vi "Autonomous Independent.vi"   [LabVIEW 2015]
doc: "This VI is called when autonomous begins, and will automatically be terminated when autonomous ends. You can carry out timed or sensor driven robot movement independently without needing to return to the caller."
uses:
  BasicAuto.ctl
  AutoPortcullis.ctl
  <vilib>/Rock Robotics/WPI/Utilities/WPI_GetSetVariantRefNum.vi
  <vilib>/Rock Robotics/Network Tables/NT Read String.vi
  <vilib>/Rock Robotics/Network Tables/NT Write Numeric Array.vi
  <vilib>/Rock Robotics/Network Tables/NT Read Numeric Array.vi
  <vilib>/Rock Robotics/Network Tables/NT Read Boolean.vi
  Robot Global Data.vi
  <vilib>/Rock Robotics/WPI/RobotDrive/WPI_RobotDriveArcadeDrive_Standard(NoSaturation).vi
types:
  T1 = typedef "WPI_JoystickDevRef.ctl" = cluster{"Device":T2}
  T2 = typedef "WPI_JoystickDeviceEnum.ctl" = enum16{"USB 0", "USB 1", "USB 2", "USB 3", "USB 4", "USB 5"}
  T3 = typedef "WPI_RobotDriveDevRef.ctl" = cluster{"DevStatus":errorcluster, "Motors[]":T4[], "Square Inputs":bool, "Max Output":dbl}
  T4 = typedef "WPI_MotorControlDeviceRef.ctl" = cluster{"DeviceStatus":errorcluster, "Type":T5, "PWM":cluster{"PWM Channel":T6, "DeadBand":T7}, "CAN":cluster{"Device Number":u8, "Control Mode":T8, "Semaphore":T9, "Max Vout":dbl, "TalonSRX Control Mode":T10}, "Invert":bool}
  T5 = typedef "WPI_MotorControlType.ctl" = enum16{"PWM", "CAN", "CANTalonSRX"}
  T6 = typedef "FPGA_DIOPWMChannel.ctl" = enum8{"PWM 0", "PWM 1", "PWM 2", "PWM 3", "PWM 4", "PWM 5", "PWM 6", "PWM 7", "PWM 8", "PWM 9", "PWM MXP 0", "PWM MXP 1", "PWM MXP 2", "PWM MXP 3", "PWM MXP 4", "PWM MXP 5", "PWM MXP 6", "PWM MXP 7", "PWM MXP 8", "PWM MXP 9", "Invalid"}
  T7 = typedef "WPI_PWMDeadband.ctl" = cluster{"Name":string, "maxPositivePwm":i32, "minPositivePwm":i32, "centerPwm":i32, "maxNegativePwm":i32, "minNegativePwm":i32, "angularRange":u16}
  T8 = typedef "WPI_CANJaguar_ControlMode.ctl" = enum8{"Percent VBus", "Current", "Speed", "Position", "Voltage"}
  T9 = typedef "Semaphore RefNum" = refnum<k1>
  T10 = typedef "WPI_CANTalonSRX_APIControlMode.ctl" = enum8{"Percent VBus", "Speed", "Position", "Slave", "Unchanged / Invalid", "Voltage Compensation", "Current", "Motion Profile"}
  T11 = typedef "WPI_DigitalInputDevRef.ctl" = cluster{"DevStatus":errorcluster, "DIO Channel":T12}
  T12 = typedef "FPGA_DIOChannel.ctl" = enum8{"DIO 0", "DIO 1", "DIO 2", "DIO 3", "DIO 4", "DIO 5", "DIO 6", "DIO 7", "DIO 8", "DIO 9", "DIO MXP 0", "DIO MXP 1", "DIO MXP 2", "DIO MXP 3", "DIO MXP 4", "DIO MXP 5", "DIO MXP 6", "DIO MXP 7", "DIO MXP 8", "DIO MXP 9", "DIO MXP 10", "DIO MXP 11", "DIO MXP 12", "DIO MXP 13", "DIO MXP 14", "DIO MXP 15", "Invalid"}
  T13 = cluster{dbl, "RobotDriveDevRef":T3, "Numeric Array":dbl[], "Boolean":bool}
  T14 = cluster{"DigitalInputDevRef":T11, "DigitalInputDevRef":T11, "MotorControlDevRef":T4}
  T15 = typedef "BasicAuto.ctl" = enum16{"Idle", "Approach", "Breach", "Travel", "Turn", "AutoTarget", "Stop"}
  T16 = typedef "AutoPortcullis.ctl" = enum16{"Idle", "Approach", "Rest", "ArmDown", "ReverseBall", "Breach", "Travel", "Stop"}
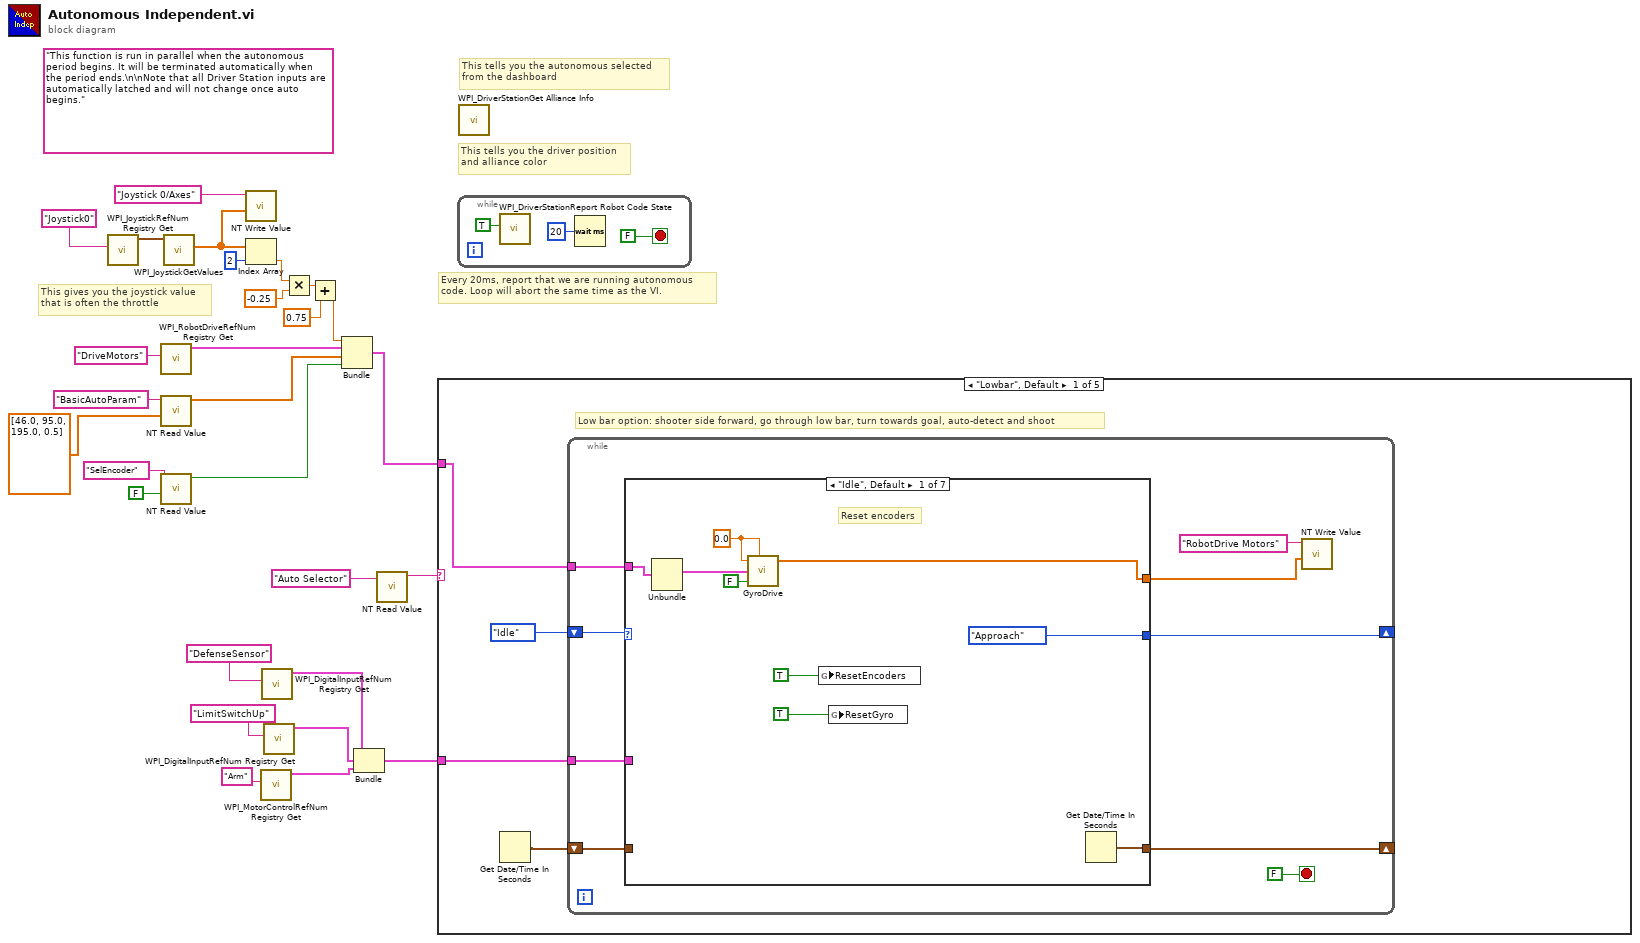
[diagram p0: block diagram]
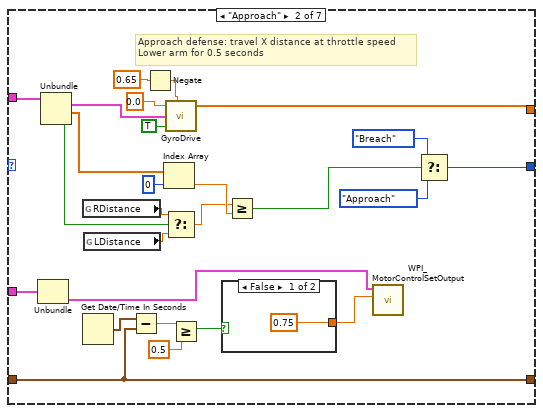
[diagram p2: hidden frame]
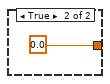
[diagram p3: hidden frame]
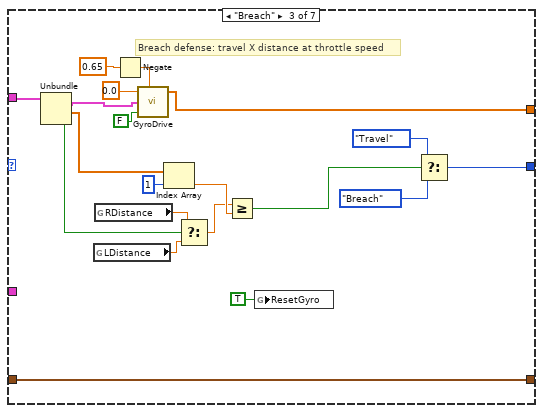
[diagram p4: hidden frame]
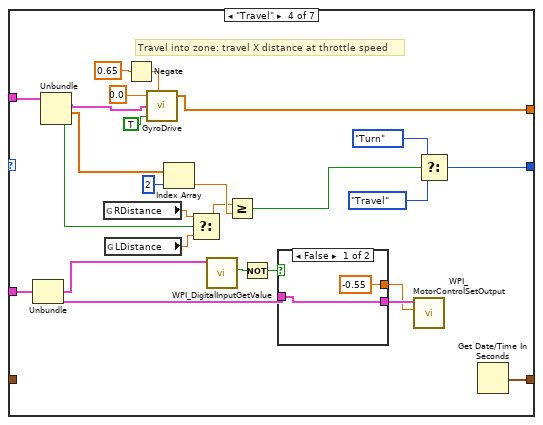
[diagram p5: hidden frame]
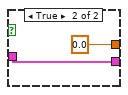
[diagram p6: hidden frame]
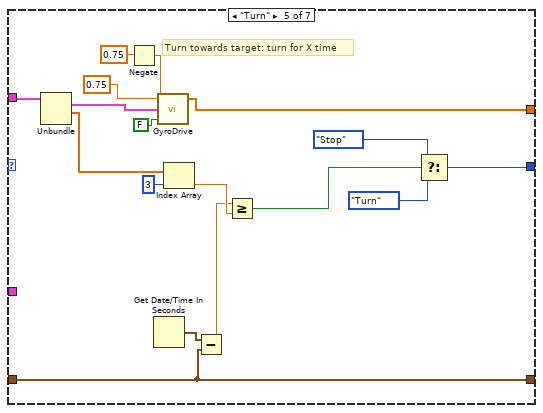
[diagram p7: hidden frame]
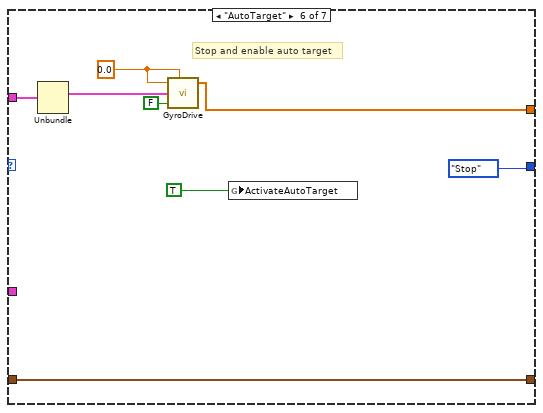
[diagram p8: hidden frame]
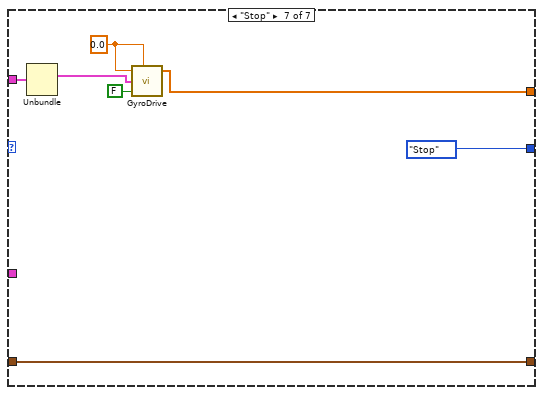
[diagram p9: hidden frame]
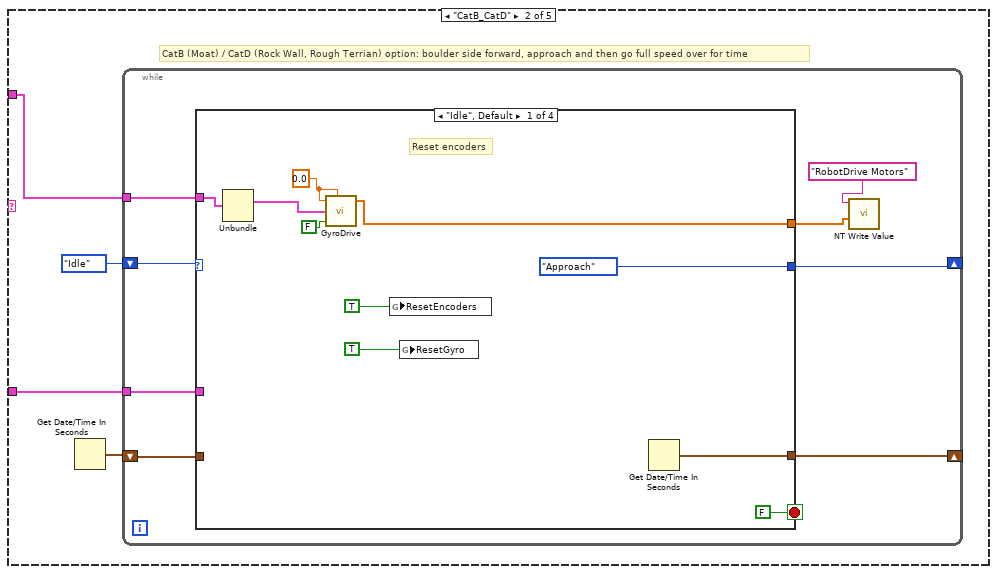
[diagram p10: hidden frame]
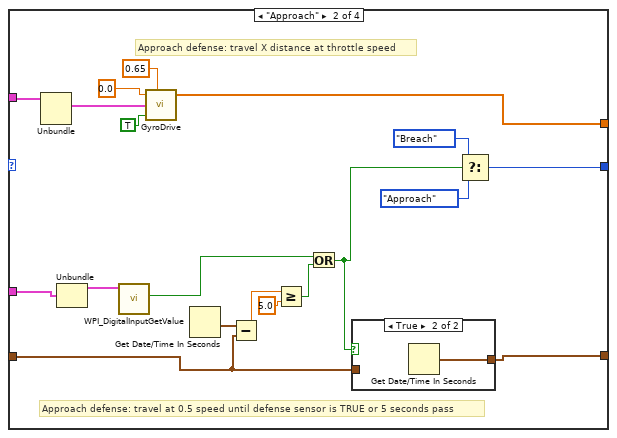
[diagram p11: hidden frame]
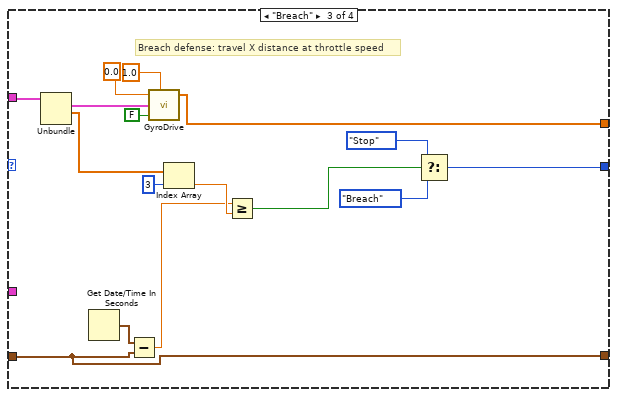
[diagram p13: hidden frame]
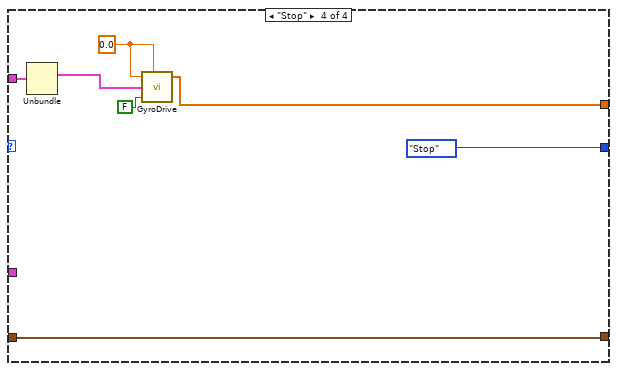
[diagram p14: hidden frame]
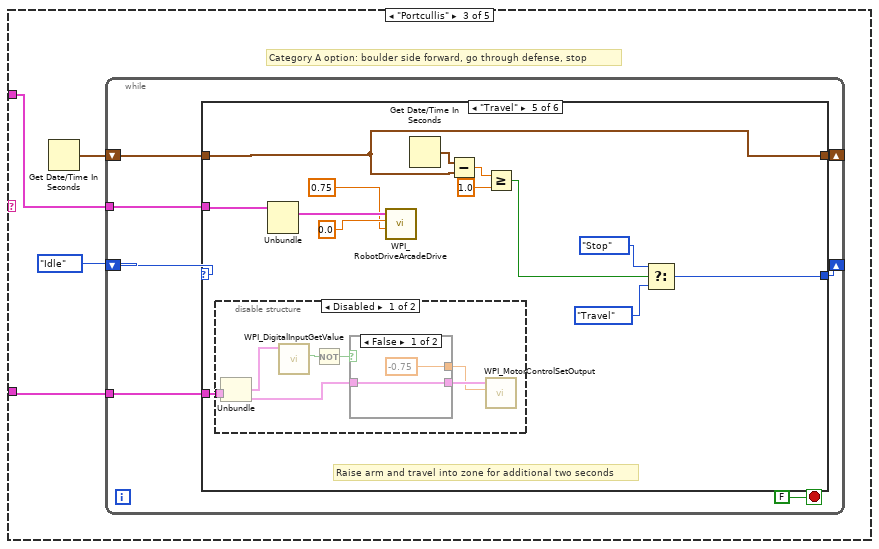
[diagram p15: hidden frame]
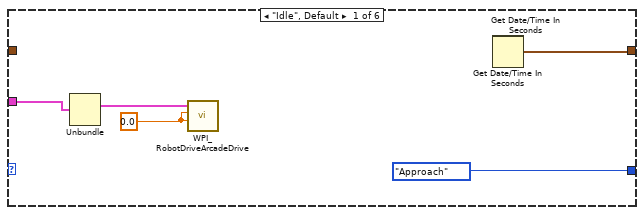
[diagram p16: hidden frame]
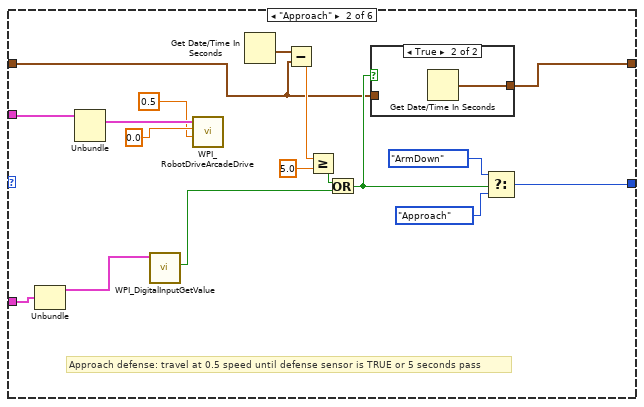
[diagram p17: hidden frame]
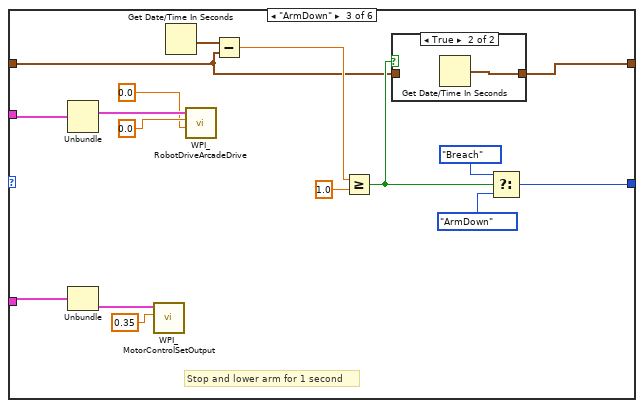
[diagram p19: hidden frame]
diagram:
  (unwired) "This function is run in parallel when the autonomous period begins. It will be terminated automatically when the period ends.\n\nNote that all Driver Station inputs are automatically latched and will not change once auto begins."
  # "This tells you the autonomous selected\nfrom the dashboard"
  # "Every 20ms, report that we are running autonomous\ncode. Loop will abort the same time as the VI."
  # "This gives you the joystick value\nthat is often the throttle"
  # "This tells you the driver position\nand alliance color"
  n1 = call <vilib>:"WPI_JoystickRefNum Registry Get.vi"("refnum name"="Joystick0") -> ("JoystickDevRef"=w27:T1)  [unwired: 1 in, 9 out]
  n2 = call <vilib>:"WPI_RobotDriveRefNum Registry Get.vi"("refnum name"="DriveMotors") -> ("RobotDriveDevRef"=w20:T3)  [unwired: 9 in, 1 out]
  n3 = call-poly <vilib>:"NT Read Value.vi"("Default Value"=dbl[] [46.0, 95.0, 195.0, 0.5], "Name"="BasicAutoParam") -> ("Numeric Array"=w17:dbl[])  [unwired: 8 in, 1 out]
  n4 = call-poly <vilib>:"NT Read Value.vi"("Default Value"=FALSE, "Name"="SelEncoder") -> ("Boolean"=w13:bool)  [unwired: 8 in, 1 out]
  n5 = call <vilib>:"WPI_JoystickGetValues.vi"("JoystickDevRef"=w27) -> ("Axes"=w23:dbl[])  [unwired: 6 in, 4 out]
  n6 = call-poly <vilib>:"NT Write Value.vi"("Numeric Array"=w23, "Name"="Joystick 0/Axes") -> ()  [unwired: 9 in, 1 out]
  n7 = Index Array(array=w23, index=2) -> (element=w9:dbl)
  n8 = call <vilib>:"WPI_MotorControlRefNum Registry Get.vi"("refnum name"="Arm") -> ("MotorControlDevRef"=w2:T4)  [unwired: 9 in, 1 out]
  n9 = call <vilib>:"WPI_DigitalInputRefNum Registry Get.vi"("refnum name"="DefenseSensor") -> ("DigitalInputDevRef"=w4:T11)  [unwired: 9 in, 1 out]
  n10 = call <vilib>:"WPI_DigitalInputRefNum Registry Get.vi"("refnum name"="LimitSwitchUp") -> ("DigitalInputDevRef"=w3:T11)  [unwired: 9 in, 1 out]
  n11 = Multiply(x=w9, y=-0.25) -> (x*y=w11:dbl)
  n12 = Add(x=w11, y=0.75) -> (x+y=w8:dbl)
  n13 = Bundle(w8, "RobotDriveDevRef"=w20, "Numeric Array"=w17, "Boolean"=w13) -> (w19:T13)  [unwired: 1 in]
  n14 = Bundle("DigitalInputDevRef"=w4, "DigitalInputDevRef"=w3, "MotorControlDevRef"=w2) -> (w1:T14)  [unwired: 1 in]
  n15 = call-poly <vilib>:"NT Read Value.vi"("Name"="Auto Selector") -> ("String"=w24:string)  [unwired: 9 in, 1 out]
  n16 = case shown="\"Lowbar\", Default" w24 {
    tunnel: w19 -> [w31 w163 w230 w327 w452]
    tunnel: w1 -> [w30 w162 w227 w324 w451]
    frame "Lowbar", Default {
      # "Low bar option: shooter side forward, go through low bar, turn towards goal, auto-detect and shoot"
      n17 = Get Date/Time In Seconds() -> (seconds since 1Jan1904=w29:timestamp)
      n18 = while {
        shift-right: [w39] -> _
        shift-left: BasicAuto."Idle" ("BasicAuto") -> [w41]
        tunnel: w31 -> [w38]
        shift-right: [w36] -> _
        shift-left: w29 -> [w37]
        tunnel: w30 -> [w35]
        stop <- FALSE stop-if-true
        n19 = case shown="\"Idle\", Default" w41 {
          tunnel: [BasicAuto."Approach" ("BasicAuto") w70 w92 w118 w139 BasicAuto."Stop" ("BasicAuto") BasicAuto."Stop" ("BasicAuto")] -> w39
          tunnel: w38 -> [w48 w76 w98 w124 w145 w152 w158]
          tunnel: [w47 w63 w86 w107 w136 w150 w159] -> w36
          tunnel: w37 -> [_ w63 w86 _ w136 w150 w159]
          tunnel: w35 -> [_ w59 _ w112 _ _ _]
          tunnel: [w44 w52 w80 w99 w129 w146 w155] -> w33
          frame "Idle", Default {
            w46 = 0.0 ("X axis value")
            # "Reset encoders"
            n20 = Unbundle(w48) -> ("RobotDriveDevRef"=w45:T3)  [unwired: 3 out]
            n21 = call "GyroDrive.vi"("X axis value"=w46, "Y axis value"=w46, "RobotDriveDevRef_In"=w45, "Use gyro"=FALSE) -> ("Motor Values"=w44:dbl[])  [unwired: 1 in, 2 out]
            n22 = global write "Robot Global Data.vi" "ResetEncoders"(TRUE) -> ()
            n23 = global write "Robot Global Data.vi" "ResetGyro"(TRUE) -> ()
            n24 = Get Date/Time In Seconds() -> (seconds since 1Jan1904=w47:timestamp)
          }
          frame "Approach" {
            # "Approach defense: travel X distance at throttle speed\nLower arm for 0.5 seconds"
            n25 = Unbundle(w59) -> ("MotorControlDevRef"=w57:T4)  [unwired: 2 out]
            n26 = Unbundle(w76) -> ("RobotDriveDevRef"=w53:T3, "Numeric Array"=w75:dbl[], "Boolean"=w68:bool)  [unwired: 1 out]
            n27 = global read "Robot Global Data.vi" "RDistance"() -> (w66:dbl)
            n28 = Get Date/Time In Seconds() -> (seconds since 1Jan1904=w64:timestamp)
            n29 = global read "Robot Global Data.vi" "LDistance"() -> (w67:dbl)
            n30 = Subtract(x=w64, y=w63) -> (x-y=w62:dbl)
            n31 = Negate(x=0.65 ("X axis value")) -> (-x=w55:dbl)
            n32 = Index Array(array=w75, index=0) -> (element=w74:dbl)
            n33 = call "GyroDrive.vi"("X axis value"=0.0, "Y axis value"=w55, "RobotDriveDevRef_In"=w53, "Use gyro"=TRUE) -> ("Motor Values"=w52:dbl[])  [unwired: 1 in, 2 out]
            n34 = Select(t=w66, s=w68, f=w67) -> (s? t:f=w65:dbl)
            n35 = Greater Or Equal?(x=w62, y=0.5) -> (x >= y?=w60:bool)
            n36 = case shown="False" w60 {
              tunnel: [0.75 0.0 ("Output")] -> w56
              frame False {
              }
              frame True {
              }
            }
            n37 = Greater Or Equal?(x=w65, y=w74) -> (x >= y?=w73:bool)
            n38 = call <vilib>:"WPI_MotorControlSetOutput.vi"("Output"=w56, "MotorControlDevRef"=w57) -> ()  [unwired: 7 in, 3 out]
            n39 = Select(t=BasicAuto."Breach" ("BasicAuto"), s=w73, f=BasicAuto."Approach" ("BasicAuto")) -> (s? t:f=w70:T15)
          }
          frame "Breach" {
            # "Breach defense: travel X distance at throttle speed"
            n40 = Unbundle(w98) -> ("RobotDriveDevRef"=w82:T3, "Numeric Array"=w97:dbl[], "Boolean"=w89:bool)  [unwired: 1 out]
            n41 = global read "Robot Global Data.vi" "LDistance"() -> (w88:dbl)
            n42 = global read "Robot Global Data.vi" "RDistance"() -> (w90:dbl)
            n43 = Negate(x=0.65 ("X axis value")) -> (-x=w84:dbl)
            n44 = call "GyroDrive.vi"("X axis value"=0.0, "Y axis value"=w84, "RobotDriveDevRef_In"=w82, "Use gyro"=FALSE) -> ("Motor Values"=w80:dbl[])  [unwired: 1 in, 2 out]
            n45 = Index Array(array=w97, index=1) -> (element=w96:dbl)
            n46 = Select(t=w90, s=w89, f=w88) -> (s? t:f=w87:dbl)
            n47 = Greater Or Equal?(x=w87, y=w96) -> (x >= y?=w95:bool)
            n48 = global write "Robot Global Data.vi" "ResetGyro"(TRUE ("ResetGyro")) -> ()
            n49 = Select(t=BasicAuto."Travel" ("BasicAuto"), s=w95, f=BasicAuto."Breach" ("BasicAuto")) -> (s? t:f=w92:T15)
          }
          frame "Travel" {
            # "Travel into zone: travel X distance at throttle speed"
            n50 = Unbundle(w112) -> ("DigitalInputDevRef"=w109:T11, "MotorControlDevRef"=w105:T4)  [unwired: 1 out]
            n51 = Unbundle(w124) -> ("RobotDriveDevRef"=w101:T3, "Numeric Array"=w123:dbl[], "Boolean"=w114:bool)  [unwired: 1 out]
            n52 = global read "Robot Global Data.vi" "RDistance"() -> (w116:dbl)
            n53 = global read "Robot Global Data.vi" "LDistance"() -> (w115:dbl)
            n54 = Negate(x=0.65 ("X axis value")) -> (-x=w103:dbl)
            n55 = call "GyroDrive.vi"("X axis value"=0.0, "Y axis value"=w103, "RobotDriveDevRef_In"=w101, "Use gyro"=TRUE) -> ("Motor Values"=w99:dbl[])  [unwired: 1 in, 2 out]
            n56 = Index Array(array=w123, index=2) -> (element=w122:dbl)
            n57 = Select(t=w116, s=w114, f=w115) -> (s? t:f=w113:dbl)
            n58 = call <vilib>:"WPI_DigitalInputGetValue.vi"("DigitalInputDevRef"=w109) -> ("Value"=w110:bool)  [unwired: 8 in, 2 out]
            n59 = Greater Or Equal?(x=w113, y=w122) -> (x >= y?=w121:bool)
            n60 = Not(x=w110) -> (.not. x?=w111:bool)
            n61 = case shown="False" w111 {
              tunnel: [w126 w128] -> w106
              tunnel: w105 -> [w126 w128]
              tunnel: [-0.55 ("Output") 0.0 ("Output")] -> w104
              frame False {
              }
              frame True {
              }
            }
            n62 = call <vilib>:"WPI_MotorControlSetOutput.vi"("Output"=w104, "MotorControlDevRef"=w106) -> ()  [unwired: 7 in, 3 out]
            n63 = Select(t=BasicAuto."Turn" ("BasicAuto"), s=w121, f=BasicAuto."Travel" ("BasicAuto")) -> (s? t:f=w118:T15)
            n64 = Get Date/Time In Seconds() -> (seconds since 1Jan1904=w107:timestamp)
          }
          frame "Turn" {
            # "Turn towards target: turn for X time"
            n65 = Unbundle(w145) -> ("RobotDriveDevRef"=w133:T3, "Numeric Array"=w144:dbl[])  [unwired: 2 out]
            n66 = Negate(x=0.75 ("y")) -> (-x=w132:dbl)
            n67 = Get Date/Time In Seconds() -> (seconds since 1Jan1904=w137:timestamp)
            n68 = call "GyroDrive.vi"("X axis value"=0.75, "Y axis value"=w132, "RobotDriveDevRef_In"=w133, "Use gyro"=FALSE) -> ("Motor Values"=w129:dbl[])  [unwired: 1 in, 2 out]
            n69 = Index Array(array=w144, index=3) -> (element=w143:dbl)
            n70 = Subtract(x=w137, y=w136) -> (x-y=w135:dbl)
            n71 = Greater Or Equal?(x=w135, y=w143) -> (x >= y?=w142:bool)
            n72 = Select(t=BasicAuto."Stop" ("BasicAuto"), s=w142, f=BasicAuto."Turn" ("BasicAuto")) -> (s? t:f=w139:T15)
          }
          frame "AutoTarget" {
            w148 = 0.0 ("X axis value")
            # "Stop and enable auto target"
            n73 = Unbundle(w152) -> ("RobotDriveDevRef"=w149:T3)  [unwired: 3 out]
            n74 = call "GyroDrive.vi"("X axis value"=w148, "Y axis value"=w148, "RobotDriveDevRef_In"=w149, "Use gyro"=FALSE) -> ("Motor Values"=w146:dbl[])  [unwired: 1 in, 2 out]
            n75 = global write "Robot Global Data.vi" "ActivateAutoTarget"(TRUE ("ActivateAutoTarget")) -> ()
          }
          frame "Stop" {
            w157 = 0.0 ("X axis value")
            n76 = Unbundle(w158) -> ("RobotDriveDevRef"=w156:T3)  [unwired: 3 out]
            n77 = call "GyroDrive.vi"("X axis value"=w157, "Y axis value"=w157, "RobotDriveDevRef_In"=w156, "Use gyro"=FALSE) -> ("Motor Values"=w155:dbl[])  [unwired: 1 in, 2 out]
          }
        }
        n78 = call-poly <vilib>:"NT Write Value.vi"("Numeric Array"=w33, "Name"="RobotDrive Motors") -> ()  [unwired: 9 in, 1 out]
      }
    }
    frame "CatB_CatD" {
      # "CatB (Moat) / CatD (Rock Wall, Rough Terrian) option: boulder side forward, approach and then go full speed over for time"
      n79 = Get Date/Time In Seconds() -> (seconds since 1Jan1904=w161:timestamp)
      n80 = while {
        shift-right: [w171] -> _
        shift-left: BasicAuto."Idle" ("BasicAuto") -> [w173]
        tunnel: w163 -> [w170]
        tunnel: w162 -> [w169]
        shift-right: [w168] -> _
        shift-left: w161 -> [w167]
        stop <- FALSE stop-if-true
        n81 = case shown="\"Idle\", Default" w173 {
          tunnel: [BasicAuto."Approach" ("BasicAuto") w198 w213 BasicAuto."Stop" ("BasicAuto")] -> w171
          tunnel: w170 -> [w180 w201 w219 w225]
          tunnel: w169 -> [_ w192 _ _]
          tunnel: [w179 w190 w210 w224] -> w168
          tunnel: w167 -> [_ w189 w210 w224]
          tunnel: [w174 w194 w205 w221] -> w165
          frame "Idle", Default {
            w176 = 0.0 ("X axis value")
            # "Reset encoders"
            n82 = Unbundle(w180) -> ("RobotDriveDevRef"=w177:T3)  [unwired: 3 out]
            n83 = call "GyroDrive.vi"("X axis value"=w176, "Y axis value"=w176, "RobotDriveDevRef_In"=w177, "Use gyro"=FALSE) -> ("Motor Values"=w174:dbl[])  [unwired: 1 in, 2 out]
            n84 = global write "Robot Global Data.vi" "ResetEncoders"(TRUE) -> ()
            n85 = global write "Robot Global Data.vi" "ResetGyro"(TRUE ("ResetGyro")) -> ()
            n86 = Get Date/Time In Seconds() -> (seconds since 1Jan1904=w179:timestamp)
          }
          frame "Approach" {
            # "Approach defense: travel at 0.5 speed until defense sensor is TRUE or 5 seconds pass"
            # "Approach defense: travel X distance at throttle speed"
            n87 = Unbundle(w201) -> ("RobotDriveDevRef"=w197:T3)  [unwired: 3 out]
            n88 = Unbundle(w192) -> ("DigitalInputDevRef"=w193:T11)  [unwired: 2 out]
            n89 = call <vilib>:"WPI_DigitalInputGetValue.vi"("DigitalInputDevRef"=w193) -> ("Value"=w186:bool)  [unwired: 8 in, 2 out]
            n90 = call "GyroDrive.vi"("X axis value"=0.0, "Y axis value"=0.65 ("X axis value"), "RobotDriveDevRef_In"=w197, "Use gyro"=TRUE) -> ("Motor Values"=w194:dbl[])  [unwired: 1 in, 2 out]
            n91 = Get Date/Time In Seconds() -> (seconds since 1Jan1904=w191:timestamp)
            n92 = Subtract(x=w191, y=w189) -> (x-y=w187:dbl)
            n93 = Greater Or Equal?(x=w187, y=5.0) -> (x >= y?=w185:bool)
            n94 = Or(x=w186, y=w185) -> (x .or. y?=w184:bool)
            n95 = case shown="True" w184 {
              tunnel: [w202 w203] -> w190
              tunnel: w189 -> [w202 _]
              frame False {
              }
              frame True {
                n96 = Get Date/Time In Seconds() -> (seconds since 1Jan1904=w203:timestamp)
              }
            }
            n97 = Select(t=BasicAuto."Breach" ("BasicAuto"), s=w184, f=BasicAuto."Approach" ("BasicAuto")) -> (s? t:f=w198:T15)
          }
          frame "Breach" {
            # "Breach defense: travel X distance at throttle speed"
            n98 = Unbundle(w219) -> ("RobotDriveDevRef"=w206:T3, "Numeric Array"=w218:dbl[])  [unwired: 2 out]
            n99 = Get Date/Time In Seconds() -> (seconds since 1Jan1904=w211:timestamp)
            n100 = Subtract(x=w211, y=w210) -> (x-y=w209:dbl)
            n101 = call "GyroDrive.vi"("X axis value"=0.0, "Y axis value"=1.0 ("X axis value"), "RobotDriveDevRef_In"=w206, "Use gyro"=FALSE) -> ("Motor Values"=w205:dbl[])  [unwired: 1 in, 2 out]
            n102 = Index Array(array=w218, index=3) -> (element=w217:dbl)
            n103 = Greater Or Equal?(x=w209, y=w217) -> (x >= y?=w216:bool)
            n104 = Select(t=BasicAuto."Stop" ("BasicAuto"), s=w216, f=BasicAuto."Breach" ("BasicAuto")) -> (s? t:f=w213:T15)
          }
          frame "Stop" {
            w223 = 0.0 ("X axis value")
            n105 = Unbundle(w225) -> ("RobotDriveDevRef"=w222:T3)  [unwired: 3 out]
            n106 = call "GyroDrive.vi"("X axis value"=w223, "Y axis value"=w223, "RobotDriveDevRef_In"=w222, "Use gyro"=FALSE) -> ("Motor Values"=w221:dbl[])  [unwired: 1 in, 2 out]
          }
        }
        n107 = call-poly <vilib>:"NT Write Value.vi"("Numeric Array"=w165, "Name"="RobotDrive Motors") -> ()  [unwired: 9 in, 1 out]
      }
    }
    frame "Portcullis" {
      # "Category A option: boulder side forward, go through defense, stop"
      n108 = Get Date/Time In Seconds() -> (seconds since 1Jan1904=w228:timestamp)
      n109 = while {
        shift-right: [w235] -> _
        shift-left: AutoPortcullis."Idle" ("AutoPortcullis") -> [w237]
        tunnel: w230 -> [w234]
        shift-right: [w232] -> _
        shift-left: w228 -> [w233]
        tunnel: w227 -> [w231]
        stop <- FALSE stop-if-true
        n110 = case shown="\"Travel\"" w237 {
          tunnel: [AutoPortcullis."Approach" ("AutoPortcullis") w257 w276 w290 w305 AutoPortcullis."Stop" ("AutoPortcullis")] -> w235
          tunnel: w234 -> [w242 w259 w268 w292 w307 w323]
          tunnel: w233 -> [_ w245 w265 w280 w299 w320]
          tunnel: [w238 w246 w267 w281 w299 w320] -> w232
          tunnel: w231 -> [_ w244 w264 _ w295 _]
          frame "Idle", Default {
            w240 = 0.0 ("X axis value")
            n111 = Unbundle(w242) -> ("RobotDriveDevRef"=w241:T3)  [unwired: 3 out]
            n112 = call-poly <vilib>:"WPI_RobotDriveArcadeDrive.vi"("Y axis value"=w240, "X axis value"=w240, "RobotDriveDevRef"=w241) -> ()  [unwired: 6 in, 3 out]
            n113 = Get Date/Time In Seconds() -> (seconds since 1Jan1904=w238:timestamp)
            n114 = Get Date/Time In Seconds() -> ()  [unwired: 1 out]
          }
          frame "Approach" {
            # "Approach defense: travel at 0.5 speed until defense sensor is TRUE or 5 seconds pass"
            n115 = Unbundle(w244) -> ("DigitalInputDevRef"=w243:T11)  [unwired: 2 out]
            n116 = Unbundle(w259) -> ("RobotDriveDevRef"=w258:T3)  [unwired: 3 out]
            n117 = call <vilib>:"WPI_DigitalInputGetValue.vi"("DigitalInputDevRef"=w243) -> ("Value"=w248:bool)  [unwired: 8 in, 2 out]
            n118 = call-poly <vilib>:"WPI_RobotDriveArcadeDrive.vi"("Y axis value"=0.5 ("X axis value"), "X axis value"=0.0, "RobotDriveDevRef"=w258) -> ()  [unwired: 6 in, 3 out]
            n119 = Get Date/Time In Seconds() -> (seconds since 1Jan1904=w252:timestamp)
            n120 = Subtract(x=w252, y=w245) -> (x-y=w251:dbl)
            n121 = Greater Or Equal?(x=w251, y=5.0) -> (x >= y?=w249:bool)
            n122 = Or(x=w249, y=w248) -> (x .or. y?=w247:bool)
            n123 = case shown="True" w247 {
              tunnel: [w260 w261] -> w246
              tunnel: w245 -> [w260 _]
              frame False {
              }
              frame True {
                n124 = Get Date/Time In Seconds() -> (seconds since 1Jan1904=w261:timestamp)
              }
            }
            n125 = Select(t=AutoPortcullis."ArmDown" ("AutoPortcullis"), s=w247, f=AutoPortcullis."Approach" ("AutoPortcullis")) -> (s? t:f=w257:T16)
          }
          frame "ArmDown" {
            # "Stop and lower arm for 1 second"
            n126 = Unbundle(w268) -> ("RobotDriveDevRef"=w271:T3)  [unwired: 3 out]
            n127 = Unbundle(w264) -> ("MotorControlDevRef"=w263:T4)  [unwired: 2 out]
            n128 = call <vilib>:"WPI_MotorControlSetOutput.vi"("Output"=0.35, "MotorControlDevRef"=w263) -> ()  [unwired: 7 in, 3 out]
            n129 = Get Date/Time In Seconds() -> (seconds since 1Jan1904=w277:timestamp)
            n130 = call-poly <vilib>:"WPI_RobotDriveArcadeDrive.vi"("Y axis value"=0.0 ("X axis value"), "X axis value"=0.0, "RobotDriveDevRef"=w271) -> ()  [unwired: 6 in, 3 out]
            n131 = Subtract(x=w277, y=w265) -> (x-y=w275:dbl)
            n132 = Greater Or Equal?(x=w275, y=1.0) -> (x >= y?=w266:bool)
            n133 = case shown="True" w266 {
              tunnel: [w278 w279] -> w267
              tunnel: w265 -> [w278 _]
              frame False {
              }
              frame True {
                n134 = Get Date/Time In Seconds() -> (seconds since 1Jan1904=w279:timestamp)
              }
            }
            n135 = Select(t=AutoPortcullis."Breach" ("AutoPortcullis"), s=w266, f=AutoPortcullis."ArmDown" ("AutoPortcullis")) -> (s? t:f=w276:T16)
          }
          frame "Breach" {
            # "Breach defense: start moving forward at higher speed"
            n136 = Unbundle(w292) -> ("RobotDriveDevRef"=w291:T3)  [unwired: 3 out]
            n137 = call-poly <vilib>:"WPI_RobotDriveArcadeDrive.vi"("Y axis value"=0.75 ("X axis value"), "X axis value"=0.0, "RobotDriveDevRef"=w291) -> ()  [unwired: 6 in, 3 out]
            n138 = Get Date/Time In Seconds() -> (seconds since 1Jan1904=w288:timestamp)
            n139 = Subtract(x=w288, y=w280) -> (x-y=w287:dbl)
            n140 = Greater Or Equal?(x=w287, y=2.0) -> (x >= y?=w282:bool)
            n141 = case shown="True" w282 {
              tunnel: [w293 w294] -> w281
              tunnel: w280 -> [w293 _]
              frame False {
              }
              frame True {
                n142 = Get Date/Time In Seconds() -> (seconds since 1Jan1904=w294:timestamp)
              }
            }
            n143 = Select(t=AutoPortcullis."Travel" ("AutoPortcullis"), s=w282, f=AutoPortcullis."Breach" ("AutoPortcullis")) -> (s? t:f=w290:T16)
          }
          frame "Travel" {
            # "Raise arm and travel into zone for additional two seconds"
            n144 = disable-structure shown="Disabled" {
              disable-tunnel: w295 -> [w312 _]
              frame Disabled {
                n145 = Unbundle(w312) -> ("DigitalInputDevRef"=w311:T11, "MotorControlDevRef"=w310:T4)  [unwired: 1 out]
                n146 = call <vilib>:"WPI_DigitalInputGetValue.vi"("DigitalInputDevRef"=w311) -> ("Value"=w313:bool)  [unwired: 8 in, 2 out]
                n147 = Not(x=w313) -> (.not. x?=w314:bool)
                n148 = case shown="False" w314 {
                  tunnel: w310 -> [w316 w318]
                  tunnel: [w316 w318] -> w309
                  tunnel: [-0.75 ("Output") 0.0 ("Output")] -> w308
                  frame False {
                  }
                  frame True {
                  }
                }
                n149 = call <vilib>:"WPI_MotorControlSetOutput.vi"("Output"=w308, "MotorControlDevRef"=w309) -> ()  [unwired: 7 in, 3 out]
              }
              frame Enabled {
              }
            }
            n150 = Unbundle(w307) -> ("RobotDriveDevRef"=w306:T3)  [unwired: 3 out]
            n151 = call-poly <vilib>:"WPI_RobotDriveArcadeDrive.vi"("Y axis value"=0.75 ("X axis value"), "X axis value"=0.0, "RobotDriveDevRef"=w306) -> ()  [unwired: 6 in, 3 out]
            n152 = Get Date/Time In Seconds() -> (seconds since 1Jan1904=w303:timestamp)
            n153 = Subtract(x=w303, y=w299) -> (x-y=w302:dbl)
            n154 = Greater Or Equal?(x=w302, y=1.0) -> (x >= y?=w300:bool)
            n155 = Select(t=AutoPortcullis."Stop" ("AutoPortcullis"), s=w300, f=AutoPortcullis."Travel" ("AutoPortcullis")) -> (s? t:f=w305:T16)
          }
          frame "Stop" {
            w321 = 0.0 ("X axis value")
            n156 = Unbundle(w323) -> ("RobotDriveDevRef"=w322:T3)  [unwired: 3 out]
            n157 = call-poly <vilib>:"WPI_RobotDriveArcadeDrive.vi"("Y axis value"=w321, "X axis value"=w321, "RobotDriveDevRef"=w322) -> ()  [unwired: 6 in, 3 out]
          }
        }
      }
    }
    frame "Cheval" {
      # "Category A option: boulder side forward, go through defense, stop"
      n158 = Get Date/Time In Seconds() -> (seconds since 1Jan1904=w325:timestamp)
      n159 = while {
        shift-right: [w334] -> _
        shift-left: AutoPortcullis."Idle" ("AutoPortcullis") -> [w336]
        tunnel: w327 -> [w333]
        shift-right: [w331] -> _
        shift-left: w325 -> [w332]
        tunnel: w324 -> [w330]
        stop <- FALSE stop-if-true
        n160 = case shown="\"Idle\", Default" w336 {
          tunnel: [AutoPortcullis."Approach" ("AutoPortcullis") w362 w378 w397 w414 w437 AutoPortcullis."Stop" ("AutoPortcullis")] -> w334
          tunnel: w333 -> [w344 w363 w379 w392 w415 w438 w449]
          tunnel: w332 -> [_ w352 w371 w389 w407 w432 w448]
          tunnel: [w342 w353 w372 w391 w408 w432 w448] -> w331
          tunnel: w330 -> [_ w351 _ w388 _ w429 _]
          tunnel: [w338 w346 w367 w383 w401 w419 w443] -> w328
          frame "Idle", Default {
            w340 = 0.0 ("X axis value")
            n161 = Unbundle(w344) -> ("RobotDriveDevRef"=w341:T3)  [unwired: 3 out]
            n162 = global write "Robot Global Data.vi" "ResetGyro"(TRUE ("ResetGyro")) -> ()
            n163 = call "GyroDrive.vi"("X axis value"=w340, "Y axis value"=w340, "RobotDriveDevRef_In"=w341, "Use gyro"=FALSE) -> ("Motor Values"=w338:dbl[])  [unwired: 1 in, 2 out]
            n164 = Get Date/Time In Seconds() -> (seconds since 1Jan1904=w342:timestamp)
            n165 = Get Date/Time In Seconds() -> ()  [unwired: 1 out]
          }
          frame "Approach" {
            # "Approach defense: travel at 0.5 speed until defense sensor is TRUE or 5 seconds pass"
            n166 = Unbundle(w351) -> ("DigitalInputDevRef"=w350:T11)  [unwired: 2 out]
            n167 = Unbundle(w363) -> ("RobotDriveDevRef"=w347:T3)  [unwired: 3 out]
            n168 = call <vilib>:"WPI_DigitalInputGetValue.vi"("DigitalInputDevRef"=w350) -> ("Value"=w355:bool)  [unwired: 8 in, 2 out]
            n169 = call "GyroDrive.vi"("X axis value"=0.0, "Y axis value"=0.55 ("X axis value"), "RobotDriveDevRef_In"=w347, "Use gyro"=TRUE) -> ("Motor Values"=w346:dbl[])  [unwired: 1 in, 2 out]
            n170 = Get Date/Time In Seconds() -> (seconds since 1Jan1904=w359:timestamp)
            n171 = Subtract(x=w359, y=w352) -> (x-y=w358:dbl)
            n172 = Greater Or Equal?(x=w358, y=5.0) -> (x >= y?=w356:bool)
            n173 = Or(x=w356, y=w355) -> (x .or. y?=w354:bool)
            n174 = case shown="True" w354 {
              tunnel: [w364 w365] -> w353
              tunnel: w352 -> [w364 _]
              frame False {
              }
              frame True {
                n175 = Get Date/Time In Seconds() -> (seconds since 1Jan1904=w365:timestamp)
              }
            }
            n176 = Select(t=AutoPortcullis."Rest" ("AutoPortcullis"), s=w354, f=AutoPortcullis."Approach" ("AutoPortcullis")) -> (s? t:f=w362:T16)
          }
          frame "Rest" {
            w368 = 0.0 ("X axis value")
            # "Rest for 0.5 seconds"
            n177 = Unbundle(w379) -> ("RobotDriveDevRef"=w369:T3)  [unwired: 3 out]
            n178 = call "GyroDrive.vi"("X axis value"=w368, "Y axis value"=w368, "RobotDriveDevRef_In"=w369, "Use gyro"=FALSE) -> ("Motor Values"=w367:dbl[])  [unwired: 1 in, 2 out]
            n179 = Get Date/Time In Seconds() -> (seconds since 1Jan1904=w375:timestamp)
            n180 = Subtract(x=w375, y=w371) -> (x-y=w374:dbl)
            n181 = Greater Or Equal?(x=w374, y=0.5) -> (x >= y?=w370:bool)
            n182 = case shown="True" w370 {
              tunnel: [w380 w381] -> w372
              tunnel: w371 -> [w380 _]
              frame False {
              }
              frame True {
                n183 = Get Date/Time In Seconds() -> (seconds since 1Jan1904=w381:timestamp)
              }
            }
            n184 = Select(t=AutoPortcullis."ArmDown" ("AutoPortcullis"), s=w370, f=AutoPortcullis."Rest" ("AutoPortcullis")) -> (s? t:f=w378:T16)
          }
          frame "ArmDown" {
            w385 = 0.0 ("X axis value")
            # "Stop and lower arm for 1 second"
            n185 = Unbundle(w392) -> ("RobotDriveDevRef"=w384:T3)  [unwired: 3 out]
            n186 = Unbundle(w388) -> ("MotorControlDevRef"=w387:T4)  [unwired: 2 out]
            n187 = call "GyroDrive.vi"("X axis value"=w385, "Y axis value"=w385, "RobotDriveDevRef_In"=w384, "Use gyro"=FALSE) -> ("Motor Values"=w383:dbl[])  [unwired: 1 in, 2 out]
            n188 = Get Date/Time In Seconds() -> (seconds since 1Jan1904=w398:timestamp)
            n189 = call <vilib>:"WPI_MotorControlSetOutput.vi"("Output"=0.75, "MotorControlDevRef"=w387) -> ()  [unwired: 7 in, 3 out]
            n190 = Subtract(x=w398, y=w389) -> (x-y=w396:dbl)
            n191 = Greater Or Equal?(x=w396, y=1.0) -> (x >= y?=w390:bool)
            n192 = case shown="True" w390 {
              tunnel: [w399 w400] -> w391
              tunnel: w389 -> [w399 _]
              frame False {
              }
              frame True {
                n193 = Get Date/Time In Seconds() -> (seconds since 1Jan1904=w400:timestamp)
              }
            }
            n194 = Select(t=AutoPortcullis."Breach" ("AutoPortcullis"), s=w390, f=AutoPortcullis."ArmDown" ("AutoPortcullis")) -> (s? t:f=w397:T16)
          }
          frame "Breach" {
            # "Breach defense: start moving forward at higher speed"
            n195 = Unbundle(w415) -> ("RobotDriveDevRef"=w405:T3)  [unwired: 3 out]
            n196 = call "GyroDrive.vi"("X axis value"=0.0, "Y axis value"=0.85 ("X axis value"), "RobotDriveDevRef_In"=w405, "Use gyro"=FALSE) -> ("Motor Values"=w401:dbl[])  [unwired: 1 in, 2 out]
            n197 = Get Date/Time In Seconds() -> (seconds since 1Jan1904=w413:timestamp)
            n198 = Subtract(x=w413, y=w407) -> (x-y=w412:dbl)
            n199 = Greater Or Equal?(x=w412, y=1.0) -> (x >= y?=w409:bool)
            n200 = case shown="True" w409 {
              tunnel: [w416 w417] -> w408
              tunnel: w407 -> [w416 _]
              frame False {
              }
              frame True {
                n201 = Get Date/Time In Seconds() -> (seconds since 1Jan1904=w417:timestamp)
              }
            }
            n202 = Select(t=AutoPortcullis."Travel" ("AutoPortcullis"), s=w409, f=AutoPortcullis."Breach" ("AutoPortcullis")) -> (s? t:f=w414:T16)
          }
          frame "Travel" {
            # "Raise arm and travel into zone for additional two seconds"
            n203 = Unbundle(w429) -> ("DigitalInputDevRef"=w423:T11, "MotorControlDevRef"=w424:T4)  [unwired: 1 out]
            n204 = Unbundle(w438) -> ("RobotDriveDevRef"=w420:T3)  [unwired: 3 out]
            n205 = call <vilib>:"WPI_DigitalInputGetValue.vi"("DigitalInputDevRef"=w423) -> ("Value"=w427:bool)  [unwired: 8 in, 2 out]
            n206 = Not(x=w427) -> (.not. x?=w428:bool)
            n207 = case shown="False" w428 {
              tunnel: w424 -> [w440 w442]
              tunnel: [w440 w442] -> w426
              tunnel: [-0.75 ("Output") 0.0 ("Output")] -> w425
              frame False {
              }
              frame True {
              }
            }
            n208 = call "GyroDrive.vi"("X axis value"=0.0, "Y axis value"=0.65 ("X axis value"), "RobotDriveDevRef_In"=w420, "Use gyro"=FALSE) -> ("Motor Values"=w419:dbl[])  [unwired: 1 in, 2 out]
            n209 = Get Date/Time In Seconds() -> (seconds since 1Jan1904=w436:timestamp)
            n210 = Subtract(x=w436, y=w432) -> (x-y=w435:dbl)
            n211 = Greater Or Equal?(x=w435, y=2.0) -> (x >= y?=w433:bool)
            n212 = call <vilib>:"WPI_MotorControlSetOutput.vi"("Output"=w425, "MotorControlDevRef"=w426) -> ()  [unwired: 7 in, 3 out]
            n213 = Select(t=AutoPortcullis."Stop" ("AutoPortcullis"), s=w433, f=AutoPortcullis."Travel" ("AutoPortcullis")) -> (s? t:f=w437:T16)
          }
          frame "Stop" {
            w445 = 0.0 ("X axis value")
            n214 = Unbundle(w449) -> ("RobotDriveDevRef"=w446:T3)  [unwired: 3 out]
            n215 = call "GyroDrive.vi"("X axis value"=w445, "Y axis value"=w445, "RobotDriveDevRef_In"=w446, "Use gyro"=FALSE) -> ("Motor Values"=w443:dbl[])  [unwired: 1 in, 2 out]
          }
        }
        n216 = call-poly <vilib>:"NT Write Value.vi"("Numeric Array"=w328, "Name"="RobotDrive Motors") -> ()  [unwired: 9 in, 1 out]
      }
    }
    frame "Approach" {
      # "Approach option: boulder side forward; approach defense until reaching ramp"
      n217 = while {
        shift-right: [w459] -> _
        shift-left: AutoPortcullis."Idle" ("AutoPortcullis") -> [w461]
        tunnel: w452 -> [w458]
        shift-right: [w456] -> _
        shift-left: _ -> [w457]
        tunnel: w451 -> [w455]
        stop <- FALSE stop-if-true
        n218 = case shown="\"Idle\", Default" w461 {
          tunnel: [AutoPortcullis."Approach" ("AutoPortcullis") w487 AutoPortcullis."Stop" ("AutoPortcullis")] -> w459
          tunnel: w458 -> [w469 w488 w497]
          tunnel: w457 -> [_ w477 w496]
          tunnel: [w467 w478 w496] -> w456
          tunnel: w455 -> [_ w476 _]
          tunnel: [w462 w470 w491] -> w453
          frame "Idle", Default {
            w465 = 0.0 ("X axis value")
            n219 = Unbundle(w469) -> ("RobotDriveDevRef"=w466:T3)  [unwired: 3 out]
            n220 = global write "Robot Global Data.vi" "ResetGyro"(TRUE) -> ()
            n221 = call "GyroDrive.vi"("X axis value"=w465, "Y axis value"=w465, "RobotDriveDevRef_In"=w466, "Use gyro"=FALSE) -> ("Motor Values"=w462:dbl[])  [unwired: 1 in, 2 out]
            n222 = Get Date/Time In Seconds() -> (seconds since 1Jan1904=w467:timestamp)
            n223 = Get Date/Time In Seconds() -> ()  [unwired: 1 out]
          }
          frame "Approach" {
            # "Approach defense: travel at 0.5 speed until defense sensor is TRUE or 5 seconds pass"
            n224 = Unbundle(w476) -> ("DigitalInputDevRef"=w475:T11)  [unwired: 2 out]
            n225 = Unbundle(w488) -> ("RobotDriveDevRef"=w472:T3)  [unwired: 3 out]
            n226 = call <vilib>:"WPI_DigitalInputGetValue.vi"("DigitalInputDevRef"=w475) -> ("Value"=w480:bool)  [unwired: 8 in, 2 out]
            n227 = call "GyroDrive.vi"("X axis value"=0.0, "Y axis value"=0.65 ("X axis value"), "RobotDriveDevRef_In"=w472, "Use gyro"=TRUE) -> ("Motor Values"=w470:dbl[])  [unwired: 1 in, 2 out]
            n228 = Get Date/Time In Seconds() -> (seconds since 1Jan1904=w484:timestamp)
            n229 = Subtract(x=w484, y=w477) -> (x-y=w483:dbl)
            n230 = Greater Or Equal?(x=w483, y=5.0) -> (x >= y?=w481:bool)
            n231 = Or(x=w481, y=w480) -> (x .or. y?=w479:bool)
            n232 = case shown="True" w479 {
              tunnel: [w489 w490] -> w478
              tunnel: w477 -> [w489 _]
              frame False {
              }
              frame True {
                n233 = Get Date/Time In Seconds() -> (seconds since 1Jan1904=w490:timestamp)
              }
            }
            n234 = Select(t=AutoPortcullis."Stop" ("AutoPortcullis"), s=w479, f=AutoPortcullis."Approach" ("AutoPortcullis")) -> (s? t:f=w487:T16)
          }
          frame "Stop" {
            w494 = 0.0
            n235 = Unbundle(w497) -> ("RobotDriveDevRef"=w493:T3)  [unwired: 3 out]
            n236 = call "GyroDrive.vi"("X axis value"=w494, "Y axis value"=w494, "RobotDriveDevRef_In"=w493, "Use gyro"=FALSE) -> ("Motor Values"=w491:dbl[])  [unwired: 1 in, 2 out]
          }
        }
        n237 = call-poly <vilib>:"NT Write Value.vi"("Numeric Array"=w453, "Name"="RobotDrive Motors") -> ()  [unwired: 9 in, 1 out]
      }
    }
  }
  n238 = while {
    stop <- FALSE stop-if-true
    n239 = call <vilib>:"WPI_DriverStationReport Robot Code State.vi"("Autonomous"=TRUE) -> ()  [unwired: 10 in, 1 out]
    n240 = Wait (ms)(milliseconds to wait=u32 20) -> ()  [unwired: 1 out]
  }
  n241 = call <vilib>:"WPI_DriverStationGet Alliance Info.vi"() -> ()  [unwired: 12 out]
